vi "test_thermistor transfer function_OLD.vi"() -> ()   [LabVIEW 2018]
uses:
  <vilib>/platform/TimedLoop/XDataNode/XDataNode.xnode
  <vilib>/Platform/TimedLoop/XDataNode/nitl_modes.ctl
  <vilib>/Platform/TimedLoop/XDataNode/XDNodeRunTimeDep.lvlib
  <vilib>/Platform/TimedLoop/XDataNode/wakeup.ctl
  <vilib>/Platform/TimedLoop/XDataNode/timing_clust.ctl
  <vilib>/rvi/FXPMathLib/FxpAdd/XNode/nifxpmath_Add.xnode
  <vilib>/rvi/FXPMathLib/FxpDiv/XNode/nifxpmath_Div.xnode
  <vilib>/rvi/FXPMathLib/sim/FxpSim.dll
  <vilib>/rvi/FXPMathLib/FxpDiv/simVIs/DllFxpDivTemp_sub.vi
  <vilib>/rvi/FXPMathLib/FxpDiv/subVIs/nifxpmath_Div_SimConfig.ctl
panel:
  out "temperature":fxp<+/-,32,16>
  in  "stop":bool
  in  "V":fxp<+,20,4>
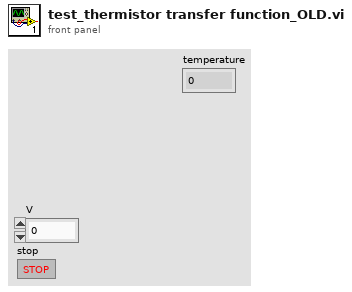
[diagram p1: front panel]
types:
  T1 = typedef "XDNodeRunTimeDep.lvlib/timing_clust.ctl" = cluster{"Expected End [f-1]":u64, "Actual End [f-1]":u64, "Finished Late? [f-1]":bool, "Expected End [i-1]":u64, "Actual End [i-1]":u64, "Finished Late? [i-1]":bool, "Expected Start [i]":u64, "Actual Start [i]":u64, "Expected Start [f]":u64, "Actual Start [f]":u64, "Source Name":string, "Structure Name":string, "Period":i64, "Deadline":i64, "Offset":i64, "Start":i64, "Priority":i32, "Timeout":i32, "Mode":T2, "Wakeup Reason":T3, "Error":errorcluster, "Source Type":string, "Secondary Source Type":string, "Global End Time":u64, "Global Start Time":u64, "Frame Duration":u64, "Iteration Duration":u64, "Assigned CPU":i32, "I/O Scan Engine Mode":u32}
  T2 = typedef "XDNodeRunTimeDep.lvlib/nitl_modes.ctl" = enum32{"No Change", "Process missed periods, maintain original phase", "Discard missed periods, maintain original phase", "Process missed periods, ignore original phase", "Discard missed periods, ignore original phase"}
  T3 = typedef "XDNodeRunTimeDep.lvlib/wakeup.ctl" = enum32{"Normal", "Aborted", "Asynchronous wakeup", "Timing source error", "Timed loop error", "Timeout"}
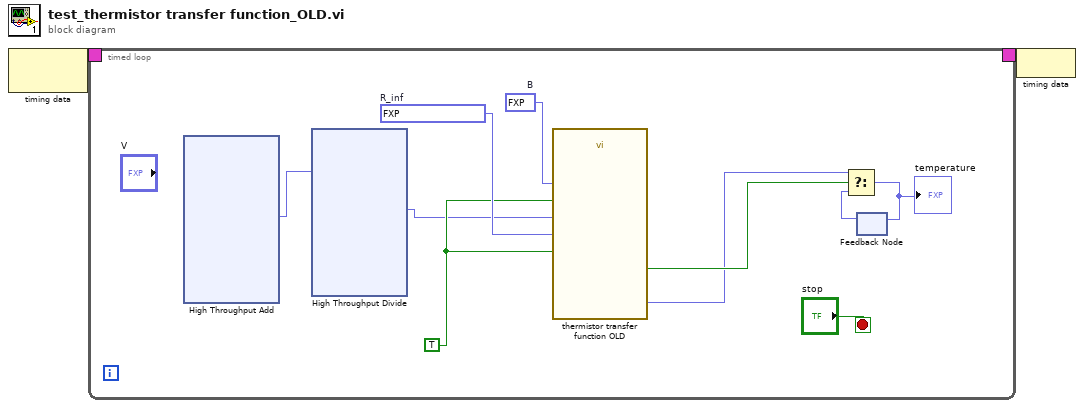
[diagram p0: block diagram]
diagram:
  n1 = node-c288() -> (w2:T1)  [unwired: 1 in]
  n2 = timed-loop {
    timing: w2 -> [_]
    timing-out: [_] -> w1
    stop <- "stop" stop-if-true
    w5 = TRUE ("input valid")
    w7 = fxp<+/-,32,16> 0.099517822265625  # R_inf
    w6 = fxp<+/-,32,16> 3434.0  # B
    n3 = xnode "High Throughput Add"() -> ("x+y"=w4:fxp<+/-,33,17>)  [unwired: 4 in, 2 out]
    n4 = xnode "High Throughput Divide"("x"=w4) -> ("x/y"=w3:fxp<+/-,32,16>)  [unwired: 3 in, 2 out]
    n5 = call "thermistor transfer function OLD.vi"("B"=w6, "R_inf"=w7, "R"=w3, "input valid"=w5, "ready for output (T)"=w5) -> ("Temperature"=w8:fxp<+/-,32,16>, "output valid"=w9:bool)  [unwired: 8 in, 1 out]
    n6 = feedback #1() -> (w11:fxp<+/-,32,16>)  [unwired: 1 in]
    n7 = Select(t=w8, s=w9, f=w11) -> (s? t:f=w12:fxp<+/-,32,16>)
    "temperature" <- w12
    n8 = feedback-in #1(w12) -> ()
  }
  n9 = node-c288(w1) -> ()
